vi "FringeScannerCloseSynchronization.vi"(2 "FringeTrackerSynchro":T1, 9 "error in (no error)":errorcluster) -> (6 "error out":errorcluster)   [LabVIEW 2009]
uses:
  Controls/FringeTrackerSynchro.ctl
  Controls/FringeScannerCommand.ctl
  Controls/FringeScannerData.ctl
  Nicmos/Controls/NICMOS.READOUT.ctl
  Controls/FringeScannerState.ctl
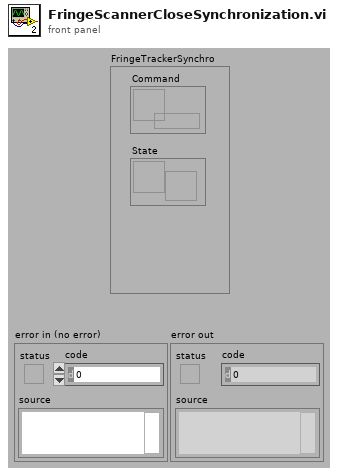
[diagram p1: front panel]
types:
  T1 = typedef "FringeTrackerSynchro.ctl" = cluster{"Command":refnum<queue>, "State":refnum<notifier>}
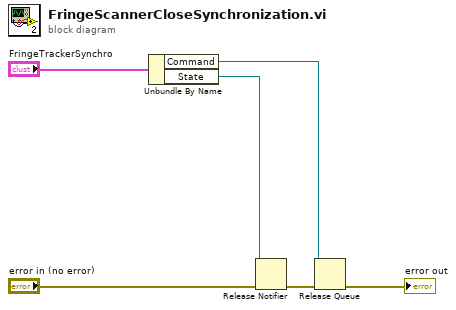
[diagram p0: block diagram]
diagram:
  n1 = Unbundle By Name("FringeTrackerSynchro") -> ("Command"=w4:refnum<queue>, "State"=w5:refnum<notifier>)
  n2 = Release Notifier(notifier=w5, error in (no error)="error in (no error)") -> (error out=w2:errorcluster)  [unwired: 1 in, 2 out]
  n3 = Release Queue(queue=w4, error in (no error)=w2) -> (error out=→"error out":errorcluster)  [unwired: 1 in, 2 out]
